vi "Drone_AUX_2.vi"(8 "error in (no error)":errorcluster, 10 "LINX Resource in":T1, 11 "AUX2":enum16{"S1", "S2", "S3", "S4"}(ring)) -> (0 "Error Out":errorcluster, 3 "LINX Resource out":T1)   [LabVIEW 2018]
uses:
  <vilib>/MakerHub/LINX/Private/Type Defs/LINX Ref.ctl
  <vilib>/MakerHub/LINX/Private/Type Defs/Platform.ctl
  <vilib>/MakerHub/LINX/Private/Type Defs/Interface.ctl
  <vilib>/MakerHub/LINX/Private/Device/Type Defs/LINX Device Config.ctl
  <vilib>/MakerHub/LINX/Private/Device/Type Defs/TCP Config.ctl
  <vilib>/MakerHub/LINX/Private/Device/Type Defs/Channels.ctl
  <vilib>/MakerHub/LINX/Public/Peripherals/Digital/Digital Write 1 Chan.vi
  <vilib>/MakerHub/LINX/Public/Peripherals/Digital/Digital Write N Chans.vi
  <vilib>/MakerHub/LINX/Private/Local IO/LinxDigitalWrite.vi
  <vilib>/MakerHub/LINX/Public/Utilities/Check Channel.vi
  <vilib>/MakerHub/LINX/Private/Utilties/Generate Error.vi
  <vilib>/MakerHub/LINX/LMH-LINX.lvlib
  <vilib>/MakerHub/LINX/Private/Device/Device.lvlib
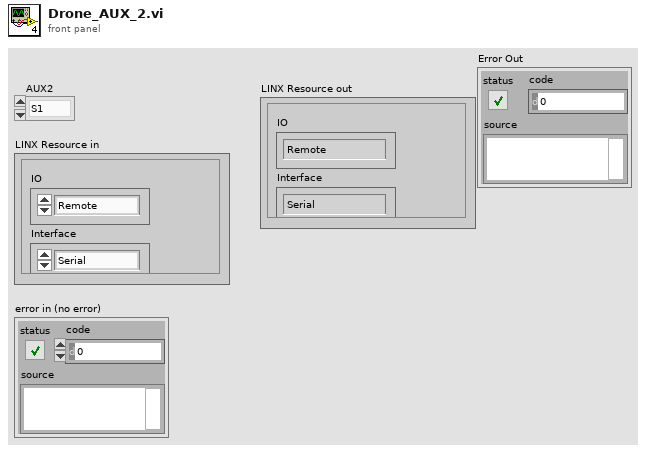
[diagram p1: front panel]
types:
  T1 = typedef "LMH-LINX.lvlib/LINX Ref.ctl" = cluster{"IO":T2, "Interface":T3, "LINX Device Config":T4}
  T2 = typedef "LMH-LINX.lvlib/Platform.ctl" = enum16{"Remote", "Local"}
  T3 = typedef "LMH-LINX.lvlib/Interface.ctl" = enum16{"Serial", "TCP"}
  T4 = typedef "LMH-LINX.lvlib/Device.lvlib/LINX Device Config.ctl" = cluster{"Interface":T3, "COM Port":refnum<visa-resource-name>, "TCP Configuration":T5, "Device Family":u8, "Device ID":u8, "Device Name":string, "TCP Ref":refnum<k5>, "Channels":T6}
  T5 = typedef "LMH-LINX.lvlib/Device.lvlib/TCP Config.ctl" = cluster{"IP Address":string, "Port":u16}
  T6 = typedef "LMH-LINX.lvlib/Channels.ctl" = cluster{"DI":u8[], "DO":u8[], "AI":u8[], "AO":u8[], "PWM":u8[], "QE":u8[], "UART":u8[], "I2C 2":u8[], "SPI":u8[], "CAN":u8[], "Servo":u8[], "AI Ref (V)":dbl, "AI Resolution (Bits)":u8, "AO Ref (V)":dbl, "AO Resolution (Bits)":u8}
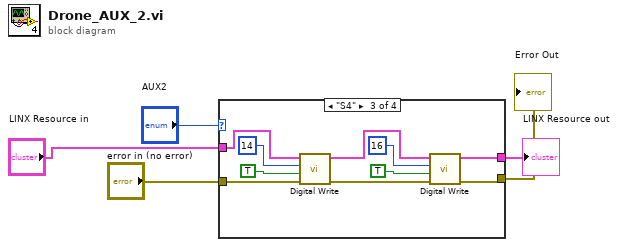
[diagram p0: block diagram]
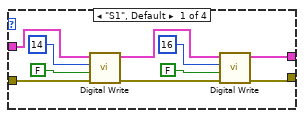
[diagram p2: hidden frame]
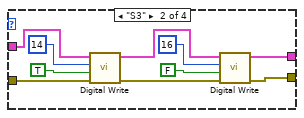
[diagram p3: hidden frame]
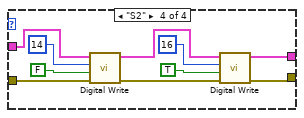
[diagram p4: hidden frame]
diagram:
  n1 = case shown="\"S4\"" "AUX2" {
    tunnel: "LINX Resource in" -> [w11 w21 w31 w41]
    tunnel: [w9 w19 w29 w39] -> w4
    tunnel: "error in (no error)" -> [w8 w18 w28 w38]
    tunnel: [w6 w16 w26 w36] -> w1
    frame "S1", Default {
      n2 = call-poly <vilib>:"Digital Write.vi"("Error In"=w8, "Output Value"=FALSE ("LED Value"), "DO Channel"=u8 14, "LINX Resource"=w11) -> ("Error Out"=w12:errorcluster, "LINX Resource"=w10:T1)  [unwired: 6 in]
      n3 = call-poly <vilib>:"Digital Write.vi"("Error In"=w12, "Output Value"=FALSE, "DO Channel"=u8 16, "LINX Resource"=w10) -> ("Error Out"=w6:errorcluster, "LINX Resource"=w9:T1)  [unwired: 6 in]
    }
    frame "S3" {
      n4 = call-poly <vilib>:"Digital Write.vi"("Error In"=w18, "Output Value"=TRUE ("LED Value"), "DO Channel"=u8 14, "LINX Resource"=w21) -> ("Error Out"=w22:errorcluster, "LINX Resource"=w20:T1)  [unwired: 6 in]
      n5 = call-poly <vilib>:"Digital Write.vi"("Error In"=w22, "Output Value"=FALSE, "DO Channel"=u8 16, "LINX Resource"=w20) -> ("Error Out"=w16:errorcluster, "LINX Resource"=w19:T1)  [unwired: 6 in]
    }
    frame "S4" {
      n6 = call-poly <vilib>:"Digital Write.vi"("Error In"=w28, "Output Value"=TRUE ("LED Value"), "DO Channel"=u8 14, "LINX Resource"=w31) -> ("Error Out"=w32:errorcluster, "LINX Resource"=w30:T1)  [unwired: 6 in]
      n7 = call-poly <vilib>:"Digital Write.vi"("Error In"=w32, "Output Value"=TRUE, "DO Channel"=u8 16, "LINX Resource"=w30) -> ("Error Out"=w26:errorcluster, "LINX Resource"=w29:T1)  [unwired: 6 in]
    }
    frame "S2" {
      n8 = call-poly <vilib>:"Digital Write.vi"("Error In"=w38, "Output Value"=FALSE ("LED Value"), "DO Channel"=u8 14, "LINX Resource"=w41) -> ("Error Out"=w42:errorcluster, "LINX Resource"=w40:T1)  [unwired: 6 in]
      n9 = call-poly <vilib>:"Digital Write.vi"("Error In"=w42, "Output Value"=TRUE, "DO Channel"=u8 16, "LINX Resource"=w40) -> ("Error Out"=w36:errorcluster, "LINX Resource"=w39:T1)  [unwired: 6 in]
    }
  }
  "LINX Resource out" <- w4
  "Error Out" <- w1
